vi "Read Msg Self.vi"(11 "Base Actor in":refnum<class "Base Actor.lvclass">) -> (2 "Msg Self":refnum<class "Msg Self.lvclass">)   [LabVIEW 2020, in "jettl.lvlib" / "Base jettl Actor.lvlib" / "Base Actor.lvlib" / "Base Actor.lvclass"]
uses:
  Base Actor.lvclass
  Base Actor.lvclass/Base Actor.ctl
  Msg Self/Msg Self.lvclass
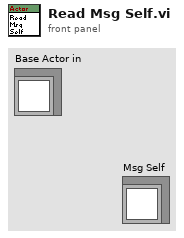
[diagram p1: front panel]
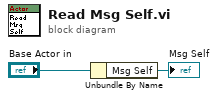
[diagram p0: block diagram]
diagram:
  n1 = Unbundle By Name("Base Actor in") -> ("Msg Self"=→"Msg Self":refnum<class "Msg Self.lvclass">)
